vi "LVCAM Create.vi"(10 "Self Actor":refnum<class "LVCAM.lvclass">, 11 "Process in":refnum<class "ABD.lvclass">) -> (0 "error out":errorcluster, 3 "Process out":refnum<class "ABD.lvclass">)   [LabVIEW 2021, in "ABD.lvlib" / "ABD.lvclass"]
uses:
  ABD.lvclass
  LVCAM/LVCAM/LVCAM/LVCAM.lvclass
  ABD.lvclass/ABD.ctl
  Open UI/Open UI Msg/Open UI Msg.lvclass
  C:/PPLs/LabVIEW-Composed-Actor-Model-LVCAM/LabVIEW-Composed-Actor-Model-LVCAM/LVCAM/LVCAM/Msg/Msg.lvclass
  LVCAM/LVCAM/Self Actor/Self Msg Send.vi
  LVCAM/LVCAM/Self Actor/Self Actor.lvclass
  C:/PPLs/LabVIEW-Composed-Actor-Model-LVCAM/LabVIEW-Composed-Actor-Model-LVCAM/Example/Open UI/Open UI Msg/Open UI Msg.lvclass
  C:/PPLs/LabVIEW-Composed-Actor-Model-LVCAM/LabVIEW-Composed-Actor-Model-LVCAM/Example/Open UI/Open UI/Open UI.lvclass
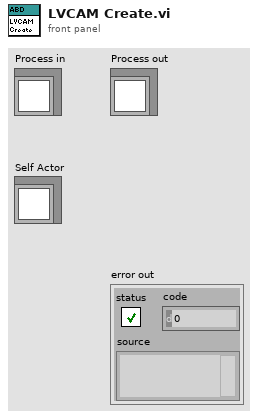
[diagram p1: front panel]
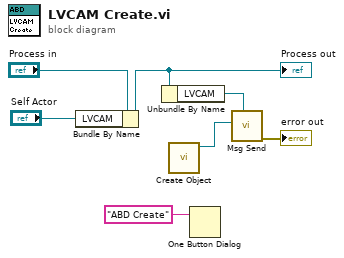
[diagram p0: block diagram]
diagram:
  n1 = Bundle By Name(cluster="Process in", "LVCAM"="Self Actor") -> (w5:refnum<class "ABD.lvclass">)
  "Process out" <- w5
  n2 = Unbundle By Name(w5) -> ("LVCAM"=w4:refnum<class "LVCAM.lvclass">)
  n3 = call "Create Object.vi"() -> ("Open UI Msg out"=w2:refnum<class "Open UI Msg.lvclass">)  [unwired: 11 in]
  n4 = One Button Dialog(message="ABD Create") -> ()  [unwired: 1 in, 1 out]
  n5 = call-poly "Msg Send.vi"("Self Actor"=w4, "Msg"=w2) -> ("error out"=→"error out":errorcluster)  [unwired: 9 in]
